vi "executePlayVSS.vi"(8 "error in (no error)":errorcluster, 11 "Game in":refnum<class "Game.lvclass">) -> (0 "error out":errorcluster, 3 "Game out":refnum<class "Game.lvclass">)   [LabVIEW 2023, in "Game.lvclass"]
uses:
  Game.lvclass
  Utilities_class/Utilities.lvclass
  Game.lvclass/Game.ctl
  Team_class/Team.lvclass/Team.ctl
  Playbook_class/Playbook.lvclass/Playbook.ctl
  HaltPlay_class/HaltPlay.lvclass/HaltPlay.ctl
  TimeoutPlay_class/TimeoutPlay.lvclass/TimeoutPlay.ctl
  PrepareFreeBallPlayVSS_class/PrepareFreeBallPlayVSS.lvclass
  PrepareGoalKickEnemyPlayVSS_class/PrepareGoalKickEnemyPlayVSS.lvclass
  PrepareGoalKickAllyPlayVSS_class/PrepareGoalKickAllyPlayVSS.lvclass
  PrepareKickoffEnemyPlay_class/PrepareKickoffEnemyPlay.lvclass
  PrepareKickoffAllyPlayVSS_class/PrepareKickoffAllyPlayVSS.lvclass
  PreparePenaltyEnemyPlayVSS_class/PreparePenaltyEnemyPlayVSS.lvclass
  PreparePenaltyAllyPlayVSS_class/PreparePenaltyAllyPlayVSS.lvclass
  Playbook_class/Read offensive_plays.vi
  HaltPlay_class/Read Roles.vi
  TimeoutPlay_class/Read Roles.vi
  Read KeeperTeam.vi
  Team_class/Read RobotRef.vi
  Team_class/Write RobotRef.vi
  Team_class/Write OffensivePlay Finished.vi
  Write KeeperTeam.vi
  Ally_class/Ally.lvclass
  C:/Users/roboi/Downloads/VSS_AI-Larc2023 - Copia (2)/Team_class/Team.lvclass
  Playbook_class/Playbook.lvclass
  Robot_class/Robot.lvclass
  Play_class/Play.lvclass
  TestPlay_class/TestPlay.lvclass
  EnemyPossessionAtEnemyFieldPlay_class/EnemyPossessionAtEnemyFieldPlay.lvclass
  EnemyPossessionAtOurFieldPlay_class/EnemyPossessionAtOurFieldPlay.lvclass
  NormalGamePlay_class/NormalGamePlay.lvclass
  IndirectEnemyPlay_class/IndirectEnemyPlay.lvclass
  PrepareKickoffAllyPlay_class/PrepareKickoffAllyPlay.lvclass
  KickPenaltyAllyPlay_class/KickPenaltyAllyPlay.lvclass
  PreparePenaltyAllyPlay_class/PreparePenaltyAllyPlay.lvclass
  DirectEnemyPlay_class/DirectEnemyPlay.lvclass
  PreparePenaltyEnemyPlay_class/PreparePenaltyEnemyPlay.lvclass
  BallOutOfFieldPlay_class/BallOutOfFieldPlay.lvclass
  StopOffensivePlay_class/StopOffensivePlay.lvclass
  PassPlay_class/PassPlay.lvclass
  DirectKickPlay_class/DirectKickPlay.lvclass
  HaltPlay_class/HaltPlay.lvclass
  PreparePassPlay_class/PreparePassPlay.lvclass
  PassToStriker_class/PassToStriker.lvclass
  PassTo2ndStriker_class/PassTo2ndStriker.lvclass
  SimplePass_class/SimplePass.lvclass
  PrepareRollToPassPlay_class/PrepareRollToPassPlay.lvclass
  PrepareDoublePassPlay_class/PrepareDoublePassPlay.lvclass
  TableWith2ndStrikerPlay_class/TableWith2ndStrikerPlay.lvclass
  TableWithStrikerPlay_class/TableWithStrikerPlay.lvclass
  HaltRole_class/HaltRole.lvclass
  DeadBallPlayVSS_class/DeadBallPlayVSS.lvclass
  NormalGamePlayVSS_class/NormalGamePlayVSS.lvclass
  BallChallengePlayVSS_class/BallChallengePlayVSS.lvclass
  PenaltyEnemyPlayVSS_class/PenaltyEnemyPlayVSS.lvclass
  TimeoutPlay_class/TimeoutPlay.lvclass
  KickPenaltyAllyPlayVSS_class/KickPenaltyAllyPlayVSS.lvclass
  PrepareKickoffEnemyPlayVSS_class/PrepareKickoffEnemyPlayVSS.lvclass
  FreeBallPlayVSS_class/FreeBallPlayVSS.lvclass
  GoalKickAllyPlayVSS_class/GoalKickAllyPlayVSS.lvclass
  GoalKickEnemyPlayVSS_class/GoalKickEnemyPlayVSS.lvclass
  KickoffAllyPlayVSS_class/KickoffAllyPlayVSS.lvclass
  KickoffEnemyPlayVSS_class/KickoffEnemyPlayVSS.lvclass
  StopPlayVSS_class/StopPlayVSS.lvclass
  AttackerAimGoalRoleVSS_class/AttackerAimGoalRoleVSS.lvclass
  BallChallengerAttackerRoleVSS_class/BallChallengerAttackerRoleVSS.lvclass
  KeeperRoleVSS_class/KeeperRoleVSS.lvclass
  NormalAttackerRoleVSS_class/NormalAttackerRoleVSS.lvclass
  DefenderAreaRoleVSS_class/DefenderAreaRoleVSS.lvclass
  GoAndKickRoleVSS_class/GoAndKickRoleVSS.lvclass
  GoalKickKeeperRoleVSS_class/GoalKickKeeperRoleVSS.lvclass
  TimeoutRole_class/TimeoutRole.lvclass
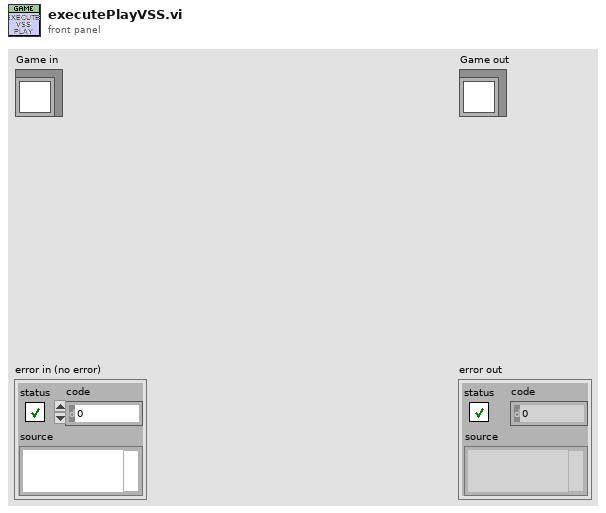
[diagram p1: front panel]
types:
  T1 = cluster{"id":i32, "x":dbl, "y":dbl, "orientation":dbl}[]
  T2 = enum16{"FreeBall", "PrepareFreeBall", "GoalKickEnemy", "GoalKickAlly", "KickoffAlly", "KickoffEnemy", "PrepareGoalKickEnemy", "PrepareGoalKickAlly", "Stop", "PrepareKickoffEnemy", "PrepareKickoffAlly", "PreparePenaltyEnemy", "Timeout", "DeadBall", "NormalGame", "KickPenaltyAlly", "PenaltyEnemy", "BallChallenge", "PreparePenaltyAlly", "Halt"}
  T3 = typedef "offensive_plays.ctl" = cluster{"Play":refnum<class "Play.lvclass">, "TestPlay":refnum<class "TestPlay.lvclass">, "EnemyPossessionAtEnemyFieldPlay":refnum<class "EnemyPossessionAtEnemyFieldPlay.lvclass">, "EnemyPossessionAtOurFieldPlay":refnum<class "EnemyPossessionAtOurFieldPlay.lvclass">, "NormalGamePlay":refnum<class "NormalGamePlay.lvclass">, "IndirectEnemyPlay":refnum<class "IndirectEnemyPlay.lvclass">, "PrepareKickoffAllyPlay":refnum<class "PrepareKickoffAllyPlay.lvclass">, "PrepareKickoffEnemyPlay":refnum<class "PrepareKickoffEnemyPlay.lvclass">, "KickPenaltyAllyPlay":refnum<class "KickPenaltyAllyPlay.lvclass">, "PreparePenaltyAllyPlay":refnum<class "PreparePenaltyAllyPlay.lvclass">, "DirectEnemyPlay":refnum<class "DirectEnemyPlay.lvclass">, "PreparePenaltyEnemyPlay":refnum<class "PreparePenaltyEnemyPlay.lvclass">, "BallOutOfFieldPlay":refnum<class "BallOutOfFieldPlay.lvclass">, "StopOffensivePlay":refnum<class "StopOffensivePlay.lvclass">, "PassPlay":refnum<class "PassPlay.lvclass">, "DirectKickPlay":refnum<class "DirectKickPlay.lvclass">, "HaltPlay":refnum<class "HaltPlay.lvclass">, "PreparePassPlay":refnum<class "PreparePassPlay.lvclass">, "PassToStrikerPlay":refnum<class "PassToStriker.lvclass">, "PassTo2ndStrikerPlay":refnum<class "PassTo2ndStriker.lvclass">, "SimplePassPlay":refnum<class "SimplePass.lvclass">, "PrepareRollToPassPlay":refnum<class "PrepareRollToPassPlay.lvclass">, "PrepareDoublePassPlay":refnum<class "PrepareDoublePassPlay.lvclass">, "TableWith2ndStrikerPlay":refnum<class "TableWith2ndStrikerPlay.lvclass">, "TableWithStrikerPlay":refnum<class "TableWithStrikerPlay.lvclass">}
  T4 = cluster{"HaltRole 1":refnum<class "HaltRole.lvclass">, "HaltRole 2":refnum<class "HaltRole.lvclass">, "HaltRole 3":refnum<class "HaltRole.lvclass">, "HaltRole 4":refnum<class "HaltRole.lvclass">, "HaltRole 5":refnum<class "HaltRole.lvclass">, "HaltRole 6":refnum<class "HaltRole.lvclass">}
  T5 = cluster{"PreparePenaltyAllyPlayVSS":refnum<class "PreparePenaltyAllyPlayVSS.lvclass">, "HaltPlay":refnum<class "HaltPlay.lvclass">, "DeadBallPlayVSS":refnum<class "DeadBallPlayVSS.lvclass">, "NormalGamePlayVSS":refnum<class "NormalGamePlayVSS.lvclass">, "BallChallengePlayVSS":refnum<class "BallChallengePlayVSS.lvclass">, "PenaltyEnemyPlayVSS":refnum<class "PenaltyEnemyPlayVSS.lvclass">, "TimeoutPlay":refnum<class "TimeoutPlay.lvclass">, "KickPenaltyAllyPlayVSS":refnum<class "KickPenaltyAllyPlayVSS.lvclass">, "PreparePenaltyEnemyPlayVSS":refnum<class "PreparePenaltyEnemyPlayVSS.lvclass">, "PrepareKickoffAllyPlayVSS":refnum<class "PrepareKickoffAllyPlayVSS.lvclass">, "PrepareKickoffEnemyPlayVSS":refnum<class "PrepareKickoffEnemyPlayVSS.lvclass">, "PrepareGoalKickAllyPlayVSS":refnum<class "PrepareGoalKickAllyPlayVSS.lvclass">, "PrepareGoalKickEnemyPlayVSS":refnum<class "PrepareGoalKickEnemyPlayVSS.lvclass">, "PrepareFreeBallPlayVSS":refnum<class "PrepareFreeBallPlayVSS.lvclass">, "FreeBallPlayVSS":refnum<class "FreeBallPlayVSS.lvclass">, "GoalKickAllyPlayVSS":refnum<class "GoalKickAllyPlayVSS.lvclass">, "GoalKickEnemyPlayVSS":refnum<class "GoalKickEnemyPlayVSS.lvclass">, "KickoffAllyPlayVSS":refnum<class "KickoffAllyPlayVSS.lvclass">, "KickoffEnemyPlayVSS":refnum<class "KickoffEnemyPlayVSS.lvclass">, "StopPlayVSS":refnum<class "StopPlayVSS.lvclass">}
  T6 = cluster{"HaltRole 1":refnum<class "HaltRole.lvclass">, "HaltRole 2":refnum<class "HaltRole.lvclass">, "AttackerAimGoalRoleVSS":refnum<class "AttackerAimGoalRoleVSS.lvclass">}
  T7 = cluster{"HaltRole 1":refnum<class "HaltRole.lvclass">, "HaltRole 2":refnum<class "HaltRole.lvclass">, "BallChallengerAttackerRoleVSS":refnum<class "BallChallengerAttackerRoleVSS.lvclass">}
  T8 = cluster{"KeeperRoleVSS":refnum<class "KeeperRoleVSS.lvclass">, "HaltRole A":refnum<class "HaltRole.lvclass">, "HaltRole D":refnum<class "HaltRole.lvclass">}
  T9 = cluster{"NormalAttackerRoleVSS":refnum<class "NormalAttackerRoleVSS.lvclass">, "HaltRole K":refnum<class "HaltRole.lvclass">, "HaltRole D":refnum<class "HaltRole.lvclass">}
  T10 = cluster{"NormalAttackerRoleVSS":refnum<class "NormalAttackerRoleVSS.lvclass">, "KeeperRoleVSS":refnum<class "KeeperRoleVSS.lvclass">, "DefenderAreaRoleVSS":refnum<class "DefenderAreaRoleVSS.lvclass">}
  T11 = cluster{"HaltRole K":refnum<class "HaltRole.lvclass">, "HaltRole D":refnum<class "HaltRole.lvclass">, "HaltRole A":refnum<class "HaltRole.lvclass">}
  T12 = cluster{"KeeperRoleVSS":refnum<class "KeeperRoleVSS.lvclass">, "HaltRole":refnum<class "HaltRole.lvclass">, "GoAndKickRoleVSS":refnum<class "GoAndKickRoleVSS.lvclass">}
  T13 = cluster{"HaltRole A":refnum<class "HaltRole.lvclass">, "HaltRole D":refnum<class "HaltRole.lvclass">, "GoalKickKeeperRoleVSS":refnum<class "GoalKickKeeperRoleVSS.lvclass">}
  T14 = cluster{"KeeperRoleVSS":refnum<class "KeeperRoleVSS.lvclass">, "DefenderAreaRoleVSS":refnum<class "DefenderAreaRoleVSS.lvclass">, "HaltRole":refnum<class "HaltRole.lvclass">}
  T15 = cluster{"TimeoutRole 1":refnum<class "TimeoutRole.lvclass">, "TimeoutRole 2":refnum<class "TimeoutRole.lvclass">, "TimeoutRole 3":refnum<class "TimeoutRole.lvclass">, "TimeoutRole 4":refnum<class "TimeoutRole.lvclass">, "TimeoutRole 5":refnum<class "TimeoutRole.lvclass">, "TimeoutRole 6":refnum<class "TimeoutRole.lvclass">}
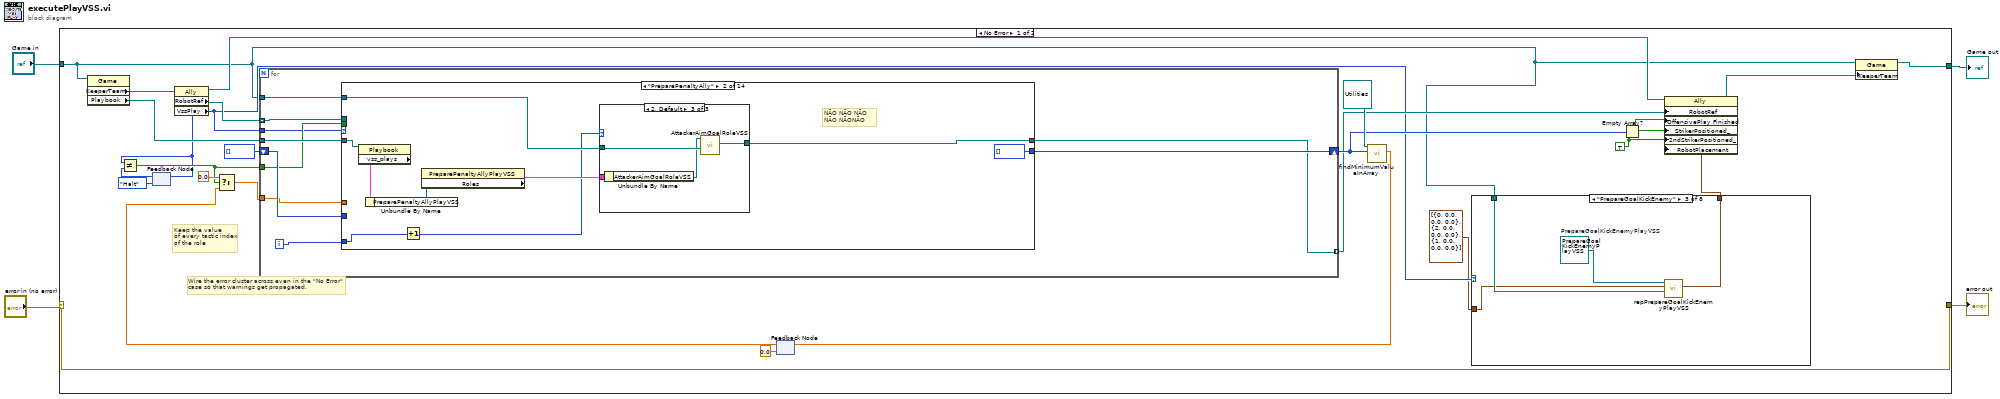
[diagram p0: block diagram]
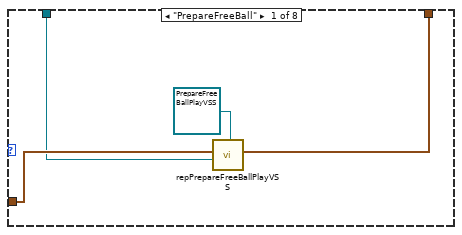
[diagram p2: hidden frame]
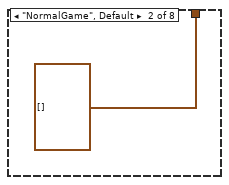
[diagram p3: hidden frame]
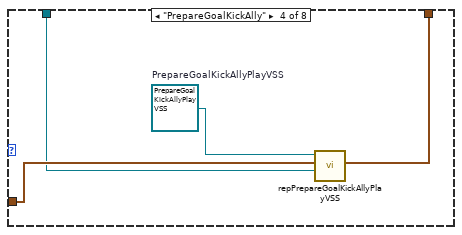
[diagram p4: hidden frame]
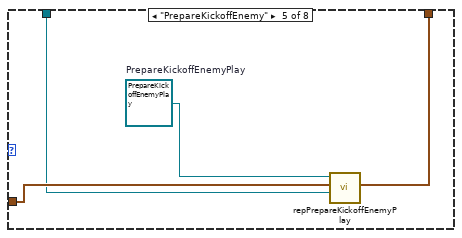
[diagram p5: hidden frame]
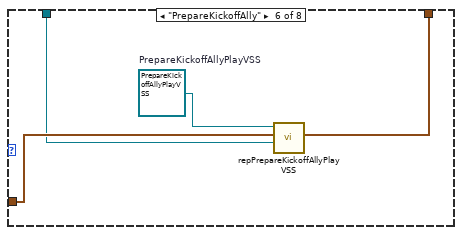
[diagram p6: hidden frame]
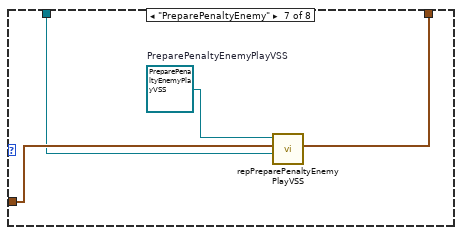
[diagram p7: hidden frame]
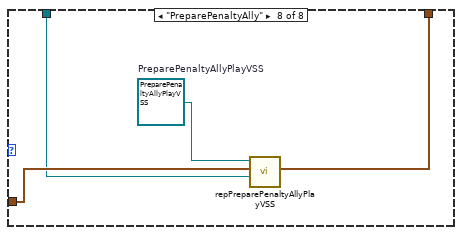
[diagram p8: hidden frame]
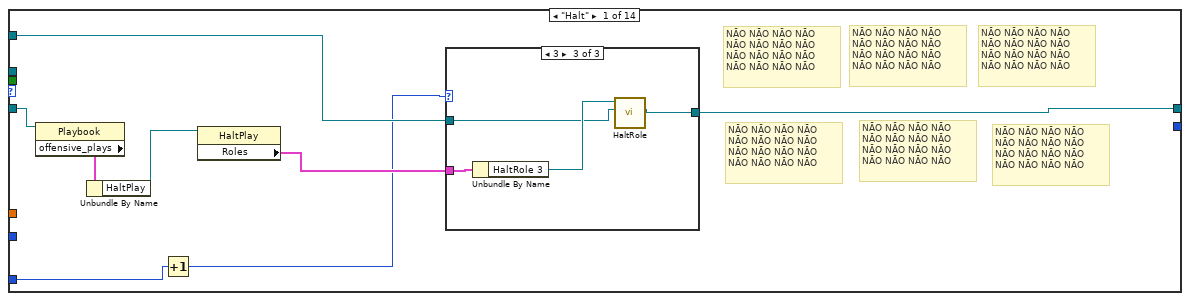
[diagram p9: hidden frame]
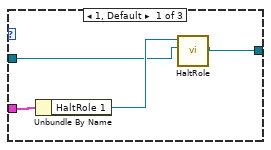
[diagram p10: hidden frame]
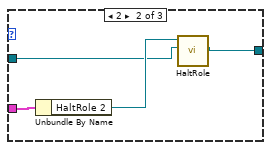
[diagram p11: hidden frame]
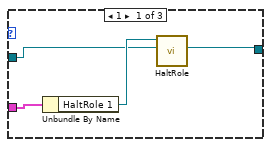
[diagram p12: hidden frame]
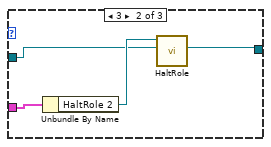
[diagram p13: hidden frame]
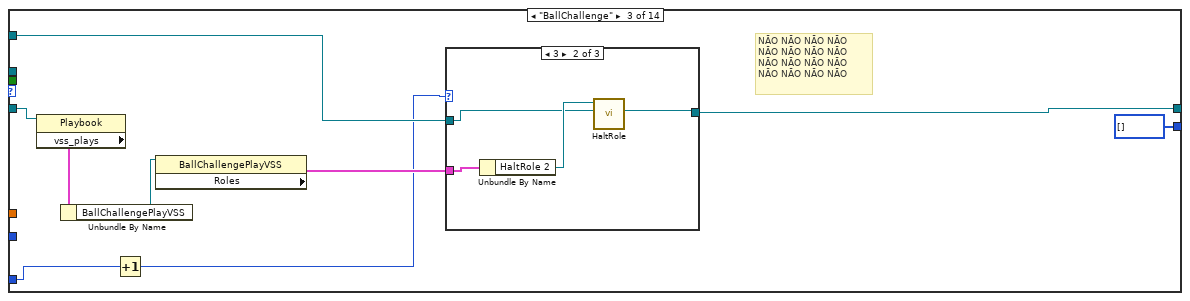
[diagram p14: hidden frame]
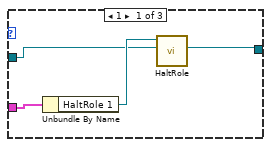
[diagram p15: hidden frame]
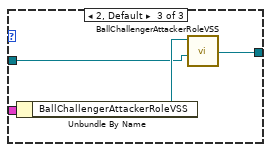
[diagram p16: hidden frame]
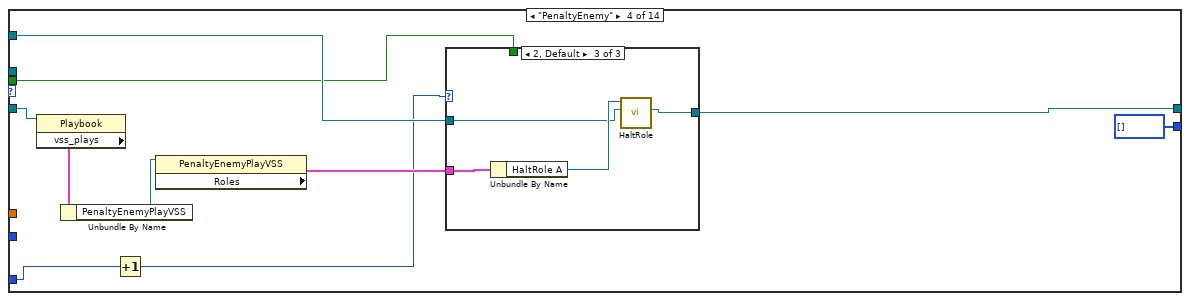
[diagram p17: hidden frame]
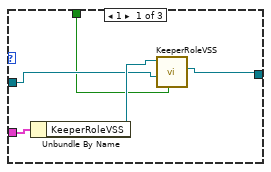
[diagram p18: hidden frame]
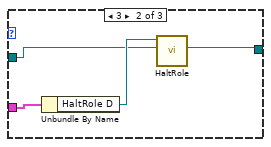
[diagram p19: hidden frame]
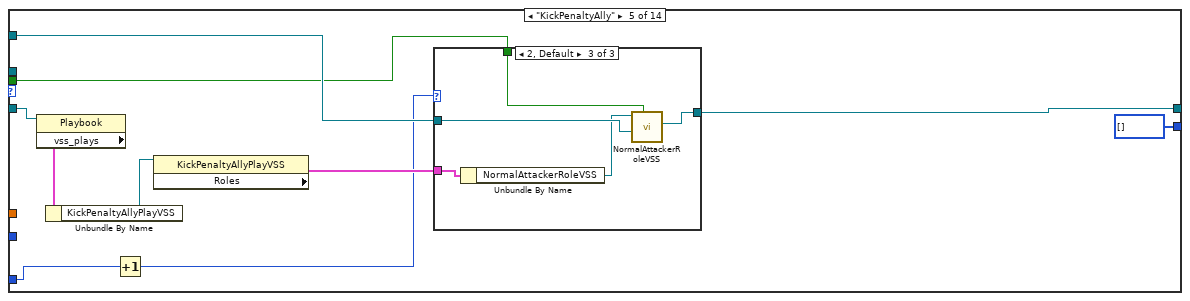
[diagram p20: hidden frame]
diagram:
  n1 = case shown="No Error" "error in (no error)" {
    selector: "error in (no error)" -> [w29 w389]
    tunnel: [w29 w389] -> w3
    tunnel: [w7 w388] -> w4
    tunnel: "Game in" -> [w8 w388]
    frame No Error {
      w14 = TRUE
      # "Keep the value\nof every tactic index\nof the role"
      # "Wire the error cluster across even in the \"No Error\"\ncase so that warnings get propagated."
      n2 = property class="Game"(reference=w8) -> ("KeeperTeam"=w28:refnum<class "Ally.lvclass">, "Playbook"=w26:refnum<class "Playbook.lvclass">)  [unwired: 1 in, 2 out]
      n3 = feedback #1(T2."Halt" ("VssPlay")) -> (w21:T2)
      n4 = property class="Ally"(reference=w28) -> (reference out=w12:refnum<class "Ally.lvclass">, "RobotRef"=w27:refnum<class "Robot.lvclass">[], "VssPlay"=w9:T2)  [unwired: 1 in, 1 out]
      n5 = Not Equal?(x=w9, y=w21) -> (x != y?=w18:bool)
      n6 = feedback-in #1(w9) -> ()
      n7 = feedback #2(0.0 ("minimum")) -> (w20:dbl)
      n8 = Select(t=0.0, s=w18, f=w20) -> (s? t:f=w13:dbl)
      n9 = for {
        tunnel: w27 -> [w63] mode=indexing
        tunnel: w26 -> [w68]
        tunnel: w8 -> [w67]
        shift-right: [w66] -> w16
        shift-left: i32[] [] -> [w65]
        tunnel: w18 -> [w64]
        tunnel: w13 -> [w62]
        tunnel: [w60] -> w11 mode=indexing
        tunnel: w9 -> [w59]
        i -> [w61]
        n10 = case shown="\"PreparePenaltyAlly\"" w59 {
          tunnel: w68 -> [w76 w97 w118 w140 w163 w186 w211 w233 w257 w280 w303 w328 w350 w372]
          tunnel: w67 -> [w72 w93 w114 w136 w159 w182 w207 w229 w253 w276 w299 w324 w346 w368]
          tunnel: [w71 w92 w113 w135 w158 w181 w206 w228 w252 w275 w298 w323 w345 w367] -> w60
          tunnel: w62 -> [_ _ _ _ _ _ _ _ _ _ _ _ _ _]
          tunnel: [_ i32[] [] i32[] [] i32[] [] i32[] [] i32[] [] i32[] [] i32[] [] i32[] [] i32[] [] i32[] [] i32[] [] i32[] [] i32[] []] -> w66
          tunnel: w65 -> [_ _ _ _ _ _ _ _ _ _ _ _ _ _]
          tunnel: w64 -> [_ _ _ w131 w154 w177 w202 w224 w248 w271 w294 w319 _ _]
          tunnel: w63 -> [_ _ _ _ _ _ _ _ _ _ _ _ _ w363]
          tunnel: w61 -> [w70 w90 w111 w133 w156 w179 w204 w226 w250 w273 w296 w321 w343 w365]
          frame "Halt" {
            # "NÃO NÃO NÃO NÃO\nNÃO NÃO NÃO NÃO\nNÃO NÃO NÃO NÃO\nNÃO NÃO NÃO NÃO"
            # "NÃO NÃO NÃO NÃO\nNÃO NÃO NÃO NÃO\nNÃO NÃO NÃO NÃO\nNÃO NÃO NÃO NÃO"
            # "NÃO NÃO NÃO NÃO\nNÃO NÃO NÃO NÃO\nNÃO NÃO NÃO NÃO\nNÃO NÃO NÃO NÃO"
            # "NÃO NÃO NÃO NÃO\nNÃO NÃO NÃO NÃO\nNÃO NÃO NÃO NÃO\nNÃO NÃO NÃO NÃO"
            # "NÃO NÃO NÃO NÃO\nNÃO NÃO NÃO NÃO\nNÃO NÃO NÃO NÃO\nNÃO NÃO NÃO NÃO"
            # "NÃO NÃO NÃO NÃO\nNÃO NÃO NÃO NÃO\nNÃO NÃO NÃO NÃO\nNÃO NÃO NÃO NÃO"
            n11 = property class="Playbook"(reference=w76) -> ("offensive_plays"=w75:T3)  [unwired: 1 in, 2 out]
            n12 = Unbundle By Name(w75) -> ("HaltPlay"=w74:refnum<class "HaltPlay.lvclass">)
            n13 = Increment(x=w70) -> (x+1=w69:i32)
            n14 = property class="HaltPlay"(reference=w74) -> ("Roles"=w73:T4)  [unwired: 1 in, 2 out]
            n15 = case shown="3" w69 {
              tunnel: w73 -> [w80 w84 w88]
              tunnel: w72 -> [w78 w82 w86]
              tunnel: [w77 w81 w85] -> w71
              frame 1, Default {
                n16 = Unbundle By Name(w80) -> ("HaltRole 1"=w79:refnum<class "HaltRole.lvclass">)
                n17 = call "HaltRole.vi"("Game in"=w78, "HaltRole in"=w79) -> ("Robot out"=w77:refnum<class "Robot.lvclass">)  [unwired: 6 in, 3 out]
              }
              frame 2 {
                n18 = Unbundle By Name(w84) -> ("HaltRole 2"=w83:refnum<class "HaltRole.lvclass">)
                n19 = call "HaltRole.vi"("Game in"=w82, "HaltRole in"=w83) -> ("Robot out"=w81:refnum<class "Robot.lvclass">)  [unwired: 6 in, 3 out]
              }
              frame 3 {
                n20 = Unbundle By Name(w88) -> ("HaltRole 3"=w87:refnum<class "HaltRole.lvclass">)
                n21 = call "HaltRole.vi"("Game in"=w86, "HaltRole in"=w87) -> ("Robot out"=w85:refnum<class "Robot.lvclass">)  [unwired: 6 in, 3 out]
              }
            }
          }
          frame "PreparePenaltyAlly" {
            # "NÃO NÃO NÃO \nNÃO NÃONÃO"
            n22 = property class="Playbook"(reference=w97) -> ("vss_plays"=w96:T5)  [unwired: 1 in, 2 out]
            n23 = Unbundle By Name(w96) -> ("PreparePenaltyAllyPlayVSS"=w95:refnum<class "PreparePenaltyAllyPlayVSS.lvclass">)
            n24 = Increment(x=w90) -> (x+1=w89:i32)
            n25 = property class="PreparePenaltyAllyPlayVSS"(reference=w95) -> ("Roles"=w94:T6)  [unwired: 1 in, 2 out]
            n26 = case shown="2, Default" w89 {
              tunnel: w94 -> [w101 w105 w109]
              tunnel: w93 -> [w99 w103 w107]
              tunnel: [w98 w102 w108] -> w92
              frame 1 {
                n27 = Unbundle By Name(w101) -> ("HaltRole 1"=w100:refnum<class "HaltRole.lvclass">)
                n28 = call "HaltRole.vi"("Game in"=w99, "HaltRole in"=w100) -> ("Robot out"=w98:refnum<class "Robot.lvclass">)  [unwired: 6 in, 3 out]
              }
              frame 3 {
                n29 = Unbundle By Name(w105) -> ("HaltRole 2"=w104:refnum<class "HaltRole.lvclass">)
                n30 = call "HaltRole.vi"("Game in"=w103, "HaltRole in"=w104) -> ("Robot out"=w102:refnum<class "Robot.lvclass">)  [unwired: 6 in, 3 out]
              }
              frame 2, Default {
                n31 = Unbundle By Name(w109) -> ("AttackerAimGoalRoleVSS"=w106:refnum<class "AttackerAimGoalRoleVSS.lvclass">)
                n32 = call "AttackerAimGoalRoleVSS.vi"("Game in"=w107, "AttackerAimGoalRoleVSS in"=w106) -> ("Robot out"=w108:refnum<class "Robot.lvclass">)  [unwired: 6 in, 3 out]
              }
            }
          }
          frame "BallChallenge" {
            # "NÃO NÃO NÃO NÃO\nNÃO NÃO NÃO NÃO\nNÃO NÃO NÃO NÃO\nNÃO NÃO NÃO NÃO"
            n33 = property class="Playbook"(reference=w118) -> ("vss_plays"=w117:T5)  [unwired: 1 in, 2 out]
            n34 = Unbundle By Name(w117) -> ("BallChallengePlayVSS"=w116:refnum<class "BallChallengePlayVSS.lvclass">)
            n35 = Increment(x=w111) -> (x+1=w110:i32)
            n36 = property class="BallChallengePlayVSS"(reference=w116) -> ("Roles"=w115:T7)  [unwired: 1 in, 2 out]
            n37 = case shown="3" w110 {
              tunnel: w115 -> [w122 w126 w130]
              tunnel: w114 -> [w120 w124 w127]
              tunnel: [w119 w123 w129] -> w113
              frame 1 {
                n38 = Unbundle By Name(w122) -> ("HaltRole 1"=w121:refnum<class "HaltRole.lvclass">)
                n39 = call "HaltRole.vi"("Game in"=w120, "HaltRole in"=w121) -> ("Robot out"=w119:refnum<class "Robot.lvclass">)  [unwired: 6 in, 3 out]
              }
              frame 3 {
                n40 = Unbundle By Name(w126) -> ("HaltRole 2"=w125:refnum<class "HaltRole.lvclass">)
                n41 = call "HaltRole.vi"("Game in"=w124, "HaltRole in"=w125) -> ("Robot out"=w123:refnum<class "Robot.lvclass">)  [unwired: 6 in, 3 out]
              }
              frame 2, Default {
                n42 = Unbundle By Name(w130) -> ("BallChallengerAttackerRoleVSS"=w128:refnum<class "BallChallengerAttackerRoleVSS.lvclass">)
                n43 = call "BallChallengerAttackerRoleVSS.vi"("Game in"=w127, "BallChallengerAttackerRoleVSS in"=w128) -> ("Robot out"=w129:refnum<class "Robot.lvclass">)  [unwired: 6 in, 3 out]
              }
            }
          }
          frame "PenaltyEnemy" {
            n44 = property class="Playbook"(reference=w140) -> ("vss_plays"=w139:T5)  [unwired: 1 in, 2 out]
            n45 = Unbundle By Name(w139) -> ("PenaltyEnemyPlayVSS"=w138:refnum<class "PenaltyEnemyPlayVSS.lvclass">)
            n46 = Increment(x=w133) -> (x+1=w132:i32)
            n47 = property class="PenaltyEnemyPlayVSS"(reference=w138) -> ("Roles"=w137:T8)  [unwired: 1 in, 2 out]
            n48 = case shown="2, Default" w132 {
              tunnel: w137 -> [w145 w149 w153]
              tunnel: w136 -> [w142 w147 w151]
              tunnel: [w144 w146 w150] -> w135
              tunnel: w131 -> [w141 _ _]
              frame 1 {
                n49 = Unbundle By Name(w145) -> ("KeeperRoleVSS"=w143:refnum<class "KeeperRoleVSS.lvclass">)
                n50 = call "KeeperRoleVSS.vi"("First call?"=w141, "Game in"=w142, "KeeperRoleVSS in"=w143) -> ("Robot out"=w144:refnum<class "Robot.lvclass">)  [unwired: 5 in, 3 out]
              }
              frame 3 {
                n51 = Unbundle By Name(w149) -> ("HaltRole D"=w148:refnum<class "HaltRole.lvclass">)
                n52 = call "HaltRole.vi"("Game in"=w147, "HaltRole in"=w148) -> ("Robot out"=w146:refnum<class "Robot.lvclass">)  [unwired: 6 in, 3 out]
              }
              frame 2, Default {
                n53 = Unbundle By Name(w153) -> ("HaltRole A"=w152:refnum<class "HaltRole.lvclass">)
                n54 = call "HaltRole.vi"("Game in"=w151, "HaltRole in"=w152) -> ("Robot out"=w150:refnum<class "Robot.lvclass">)  [unwired: 6 in, 3 out]
              }
            }
          }
          frame "KickPenaltyAlly" {
            n55 = property class="Playbook"(reference=w163) -> ("vss_plays"=w162:T5)  [unwired: 1 in, 2 out]
            n56 = Unbundle By Name(w162) -> ("KickPenaltyAllyPlayVSS"=w161:refnum<class "KickPenaltyAllyPlayVSS.lvclass">)
            n57 = Increment(x=w156) -> (x+1=w155:i32)
            n58 = property class="KickPenaltyAllyPlayVSS"(reference=w161) -> ("Roles"=w160:T9)  [unwired: 1 in, 2 out]
            n59 = case shown="2, Default" w155 {
              tunnel: w160 -> [w167 w171 w176]
              tunnel: w159 -> [w165 w169 w174]
              tunnel: [w164 w168 w172] -> w158
              tunnel: w154 -> [_ _ w175]
              frame 1 {
                n60 = Unbundle By Name(w167) -> ("HaltRole K"=w166:refnum<class "HaltRole.lvclass">)
                n61 = call "HaltRole.vi"("Game in"=w165, "HaltRole in"=w166) -> ("Robot out"=w164:refnum<class "Robot.lvclass">)  [unwired: 6 in, 3 out]
              }
              frame 3 {
                n62 = Unbundle By Name(w171) -> ("HaltRole D"=w170:refnum<class "HaltRole.lvclass">)
                n63 = call "HaltRole.vi"("Game in"=w169, "HaltRole in"=w170) -> ("Robot out"=w168:refnum<class "Robot.lvclass">)  [unwired: 6 in, 3 out]
              }
              frame 2, Default {
                n64 = Unbundle By Name(w176) -> ("NormalAttackerRoleVSS"=w173:refnum<class "NormalAttackerRoleVSS.lvclass">)
                n65 = call "NormalAttackerRoleVSS.vi"("First call?"=w175, "Game in"=w174, "NormalAttackerRoleVSS in"=w173) -> ("Robot out"=w172:refnum<class "Robot.lvclass">)  [unwired: 5 in, 3 out]
              }
            }
          }
          frame "NormalGame", Default {
            n66 = property class="Playbook"(reference=w186) -> ("vss_plays"=w185:T5)  [unwired: 1 in, 2 out]
            n67 = Unbundle By Name(w185) -> ("NormalGamePlayVSS"=w184:refnum<class "NormalGamePlayVSS.lvclass">)
            n68 = Increment(x=w179) -> (x+1=w178:i32)
            n69 = property class="NormalGamePlayVSS"(reference=w184) -> ("Roles"=w183:T10)  [unwired: 1 in, 2 out]
            n70 = case shown="2" w178 {
              tunnel: w183 -> [w191 w196 w201]
              tunnel: w182 -> [w189 w194 w199]
              tunnel: [w188 w193 w198] -> w181
              tunnel: w177 -> [w187 w192 w197]
              frame 1, Default {
                n71 = Unbundle By Name(w191) -> ("KeeperRoleVSS"=w190:refnum<class "KeeperRoleVSS.lvclass">)
                n72 = call "KeeperRoleVSS.vi"("First call?"=w187, "Game in"=w189, "KeeperRoleVSS in"=w190) -> ("Robot out"=w188:refnum<class "Robot.lvclass">)  [unwired: 5 in, 3 out]
              }
              frame 2 {
                n73 = Unbundle By Name(w196) -> ("NormalAttackerRoleVSS"=w195:refnum<class "NormalAttackerRoleVSS.lvclass">)
                n74 = call "NormalAttackerRoleVSS.vi"("First call?"=w192, "Game in"=w194, "NormalAttackerRoleVSS in"=w195) -> ("Robot out"=w193:refnum<class "Robot.lvclass">)  [unwired: 5 in, 3 out]
              }
              frame 3 {
                n75 = Unbundle By Name(w201) -> ("DefenderAreaRoleVSS"=w200:refnum<class "DefenderAreaRoleVSS.lvclass">)
                n76 = call "DefenderAreaRoleVSS.vi"("First call?"=w197, "Game in"=w199, "DefenderAreaRoleVSS in"=w200) -> ("Robot out"=w198:refnum<class "Robot.lvclass">)  [unwired: 5 in, 3 out]
              }
            }
          }
          frame "Stop" {
            n77 = property class="Playbook"(reference=w211) -> ("vss_plays"=w210:T5)  [unwired: 1 in, 2 out]
            n78 = Unbundle By Name(w210) -> ("StopPlayVSS"=w209:refnum<class "StopPlayVSS.lvclass">)
            n79 = Increment(x=w204) -> (x+1=w203:i32)
            n80 = property class="StopPlayVSS"(reference=w209) -> ("Roles"=w208:T11)  [unwired: 1 in, 2 out]
            n81 = case shown="2" w203 {
              tunnel: w208 -> [w215 w219 w223]
              tunnel: w207 -> [w214 w218 w222]
              tunnel: [w212 w216 w220] -> w206
              tunnel: w202 -> [_ _ _]
              frame 1, Default {
                n82 = Unbundle By Name(w215) -> ("HaltRole K"=w213:refnum<class "HaltRole.lvclass">)
                n83 = call "HaltRole.vi"("Game in"=w214, "HaltRole in"=w213) -> ("Robot out"=w212:refnum<class "Robot.lvclass">)  [unwired: 6 in, 3 out]
              }
              frame 3 {
                n84 = Unbundle By Name(w219) -> ("HaltRole D"=w217:refnum<class "HaltRole.lvclass">)
                n85 = call "HaltRole.vi"("Game in"=w218, "HaltRole in"=w217) -> ("Robot out"=w216:refnum<class "Robot.lvclass">)  [unwired: 6 in, 3 out]
              }
              frame 2 {
                n86 = Unbundle By Name(w223) -> ("HaltRole A"=w221:refnum<class "HaltRole.lvclass">)
                n87 = call "HaltRole.vi"("Game in"=w222, "HaltRole in"=w221) -> ("Robot out"=w220:refnum<class "Robot.lvclass">)  [unwired: 6 in, 3 out]
              }
            }
          }
          frame "KickoffAlly" {
            n88 = property class="Playbook"(reference=w233) -> ("vss_plays"=w232:T5)  [unwired: 1 in, 2 out]
            n89 = Unbundle By Name(w232) -> ("KickoffAllyPlayVSS"=w231:refnum<class "KickoffAllyPlayVSS.lvclass">)
            n90 = Increment(x=w226) -> (x+1=w225:i32)
            n91 = property class="KickoffAllyPlayVSS"(reference=w231) -> ("Roles"=w230:T12)  [unwired: 1 in, 2 out]
            n92 = case shown="2" w225 {
              tunnel: w230 -> [w238 w242 w247]
              tunnel: w229 -> [w236 w241 w245]
              tunnel: [w235 w239 w243] -> w228
              tunnel: w224 -> [w234 _ w246]
              frame 1, Default {
                n93 = Unbundle By Name(w238) -> ("KeeperRoleVSS"=w237:refnum<class "KeeperRoleVSS.lvclass">)
                n94 = call "KeeperRoleVSS.vi"("First call?"=w234, "Game in"=w236, "KeeperRoleVSS in"=w237) -> ("Robot out"=w235:refnum<class "Robot.lvclass">)  [unwired: 5 in, 3 out]
              }
              frame 3 {
                n95 = Unbundle By Name(w242) -> ("HaltRole"=w240:refnum<class "HaltRole.lvclass">)
                n96 = call "HaltRole.vi"("Game in"=w241, "HaltRole in"=w240) -> ("Robot out"=w239:refnum<class "Robot.lvclass">)  [unwired: 6 in, 3 out]
              }
              frame 2 {
                n97 = Unbundle By Name(w247) -> ("GoAndKickRoleVSS"=w244:refnum<class "GoAndKickRoleVSS.lvclass">)
                n98 = call "GoAndKickRoleVSS.vi"("First call?"=w246, "Game in"=w245, "GoAndKickRoleVSS in"=w244) -> ("Robot out"=w243:refnum<class "Robot.lvclass">)  [unwired: 5 in, 3 out]
              }
            }
          }
          frame "KickoffEnemy" {
            n99 = property class="Playbook"(reference=w257) -> ("vss_plays"=w256:T5)  [unwired: 1 in, 2 out]
            n100 = Unbundle By Name(w256) -> ("KickoffEnemyPlayVSS"=w255:refnum<class "KickoffEnemyPlayVSS.lvclass">)
            n101 = Increment(x=w250) -> (x+1=w249:i32)
            n102 = property class="KickoffEnemyPlayVSS"(reference=w255) -> ("Roles"=w254:T8)  [unwired: 1 in, 2 out]
            n103 = case shown="2" w249 {
              tunnel: w254 -> [w262 w266 w270]
              tunnel: w253 -> [w260 w265 w269]
              tunnel: [w259 w264 w267] -> w252
              tunnel: w248 -> [w258 _ _]
              frame 1, Default {
                n104 = Unbundle By Name(w262) -> ("KeeperRoleVSS"=w261:refnum<class "KeeperRoleVSS.lvclass">)
                n105 = call "KeeperRoleVSS.vi"("First call?"=w258, "Game in"=w260, "KeeperRoleVSS in"=w261) -> ("Robot out"=w259:refnum<class "Robot.lvclass">)  [unwired: 5 in, 3 out]
              }
              frame 3 {
                n106 = Unbundle By Name(w266) -> ("HaltRole D"=w263:refnum<class "HaltRole.lvclass">)
                n107 = call "HaltRole.vi"("Game in"=w265, "HaltRole in"=w263) -> ("Robot out"=w264:refnum<class "Robot.lvclass">)  [unwired: 6 in, 3 out]
              }
              frame 2 {
                n108 = Unbundle By Name(w270) -> ("HaltRole A"=w268:refnum<class "HaltRole.lvclass">)
                n109 = call "HaltRole.vi"("Game in"=w269, "HaltRole in"=w268) -> ("Robot out"=w267:refnum<class "Robot.lvclass">)  [unwired: 6 in, 3 out]
              }
            }
          }
          frame "GoalKickAlly" {
            n110 = property class="Playbook"(reference=w280) -> ("vss_plays"=w279:T5)  [unwired: 1 in, 2 out]
            n111 = Unbundle By Name(w279) -> ("GoalKickAllyPlayVSS"=w278:refnum<class "GoalKickAllyPlayVSS.lvclass">)
            n112 = Increment(x=w273) -> (x+1=w272:i32)
            n113 = property class="GoalKickAllyPlayVSS"(reference=w278) -> ("Roles"=w277:T13)  [unwired: 1 in, 2 out]
            n114 = case shown="2" w272 {
              tunnel: w277 -> [w285 w289 w293]
              tunnel: w276 -> [w282 w288 w292]
              tunnel: [w284 w287 w290] -> w275
              tunnel: w271 -> [w281 _ _]
              frame 1, Default {
                n115 = Unbundle By Name(w285) -> ("GoalKickKeeperRoleVSS"=w283:refnum<class "GoalKickKeeperRoleVSS.lvclass">)
                n116 = call "GoalKickKeeperRoleVSS.vi"("First call?"=w281, "Game in"=w282, "GoalKickKeeperRoleVSS in"=w283) -> ("Robot out"=w284:refnum<class "Robot.lvclass">)  [unwired: 5 in, 3 out]
              }
              frame 3 {
                n117 = Unbundle By Name(w289) -> ("HaltRole D"=w286:refnum<class "HaltRole.lvclass">)
                n118 = call "HaltRole.vi"("Game in"=w288, "HaltRole in"=w286) -> ("Robot out"=w287:refnum<class "Robot.lvclass">)  [unwired: 6 in, 3 out]
              }
              frame 2 {
                n119 = Unbundle By Name(w293) -> ("HaltRole A"=w291:refnum<class "HaltRole.lvclass">)
                n120 = call "HaltRole.vi"("Game in"=w292, "HaltRole in"=w291) -> ("Robot out"=w290:refnum<class "Robot.lvclass">)  [unwired: 6 in, 3 out]
              }
            }
          }
          frame "FreeBall" {
            n121 = property class="Playbook"(reference=w303) -> ("vss_plays"=w302:T5)  [unwired: 1 in, 2 out]
            n122 = Unbundle By Name(w302) -> ("FreeBallPlayVSS"=w301:refnum<class "FreeBallPlayVSS.lvclass">)
            n123 = Increment(x=w296) -> (x+1=w295:i32)
            n124 = property class="FreeBallPlayVSS"(reference=w301) -> ("Roles"=w300:T10)  [unwired: 1 in, 2 out]
            n125 = case shown="1, Default" w295 {
              tunnel: w300 -> [w308 w313 w318]
              tunnel: w299 -> [w306 w311 w316]
              tunnel: [w305 w310 w315] -> w298
              tunnel: w294 -> [w304 w309 w314]
              frame 1, Default {
                n126 = Unbundle By Name(w308) -> ("KeeperRoleVSS"=w307:refnum<class "KeeperRoleVSS.lvclass">)
                n127 = call "KeeperRoleVSS.vi"("First call?"=w304, "Game in"=w306, "KeeperRoleVSS in"=w307) -> ("Robot out"=w305:refnum<class "Robot.lvclass">)  [unwired: 5 in, 3 out]
              }
              frame 3 {
                n128 = Unbundle By Name(w313) -> ("DefenderAreaRoleVSS"=w312:refnum<class "DefenderAreaRoleVSS.lvclass">)
                n129 = call "DefenderAreaRoleVSS.vi"("First call?"=w309, "Game in"=w311, "DefenderAreaRoleVSS in"=w312) -> ("Robot out"=w310:refnum<class "Robot.lvclass">)  [unwired: 5 in, 3 out]
              }
              frame 2 {
                n130 = Unbundle By Name(w318) -> ("NormalAttackerRoleVSS"=w317:refnum<class "NormalAttackerRoleVSS.lvclass">)
                n131 = call "NormalAttackerRoleVSS.vi"("First call?"=w314, "Game in"=w316, "NormalAttackerRoleVSS in"=w317) -> ("Robot out"=w315:refnum<class "Robot.lvclass">)  [unwired: 5 in, 3 out]
              }
            }
          }
          frame "GoalKickEnemy" {
            n132 = property class="Playbook"(reference=w328) -> ("vss_plays"=w327:T5)  [unwired: 1 in, 2 out]
            n133 = Unbundle By Name(w327) -> ("GoalKickEnemyPlayVSS"=w326:refnum<class "GoalKickEnemyPlayVSS.lvclass">)
            n134 = Increment(x=w321) -> (x+1=w320:i32)
            n135 = property class="GoalKickEnemyPlayVSS"(reference=w326) -> ("Roles"=w325:T14)  [unwired: 1 in, 2 out]
            n136 = case shown="3" w320 {
              tunnel: w325 -> [w332 w337 w341]
              tunnel: w324 -> [w330 w335 w339]
              tunnel: [w329 w333 w338] -> w323
              tunnel: w319 -> [_ w336 _]
              frame 1, Default {
                n137 = Unbundle By Name(w332) -> ("KeeperRoleVSS"=w331:refnum<class "KeeperRoleVSS.lvclass">)
                n138 = call "KeeperRoleVSS.vi"("Game in"=w330, "KeeperRoleVSS in"=w331) -> ("Robot out"=w329:refnum<class "Robot.lvclass">)  [unwired: 6 in, 3 out]
              }
              frame 3 {
                n139 = Unbundle By Name(w337) -> ("DefenderAreaRoleVSS"=w334:refnum<class "DefenderAreaRoleVSS.lvclass">)
                n140 = call "DefenderAreaRoleVSS.vi"("First call?"=w336, "Game in"=w335, "DefenderAreaRoleVSS in"=w334) -> ("Robot out"=w333:refnum<class "Robot.lvclass">)  [unwired: 5 in, 3 out]
              }
              frame 2 {
                n141 = Unbundle By Name(w341) -> ("HaltRole"=w340:refnum<class "HaltRole.lvclass">)
                n142 = call "HaltRole.vi"("Game in"=w339, "HaltRole in"=w340) -> ("Robot out"=w338:refnum<class "Robot.lvclass">)  [unwired: 6 in, 3 out]
              }
            }
          }
          frame "DeadBall" {
            # "NÃO NÃO NÃO NÃO\nNÃO NÃO NÃO NÃO\nNÃO NÃO NÃO NÃO\nNÃO NÃO NÃO NÃO"
            n143 = property class="Playbook"(reference=w350) -> ("vss_plays"=w349:T5)  [unwired: 1 in, 2 out]
            n144 = Unbundle By Name(w349) -> ("DeadBallPlayVSS"=w348:refnum<class "DeadBallPlayVSS.lvclass">)
            n145 = Increment(x=w343) -> (x+1=w342:i32)
            n146 = property class="DeadBallPlayVSS"(reference=w348) -> ("Roles"=w347:T10)  [unwired: 1 in, 2 out]
            n147 = case shown="3" w342 {
              tunnel: w347 -> [w354 w358 w362]
              tunnel: w346 -> [w352 w356 w360]
              tunnel: [w351 w355 w359] -> w345
              frame 1 {
                n148 = Unbundle By Name(w354) -> ("KeeperRoleVSS"=w353:refnum<class "KeeperRoleVSS.lvclass">)
                n149 = call "KeeperRoleVSS.vi"("Game in"=w352, "KeeperRoleVSS in"=w353) -> ("Robot out"=w351:refnum<class "Robot.lvclass">)  [unwired: 6 in, 3 out]
              }
              frame 3 {
                n150 = Unbundle By Name(w358) -> ("DefenderAreaRoleVSS"=w357:refnum<class "DefenderAreaRoleVSS.lvclass">)
                n151 = call "DefenderAreaRoleVSS.vi"("Game in"=w356, "DefenderAreaRoleVSS in"=w357) -> ("Robot out"=w355:refnum<class "Robot.lvclass">)  [unwired: 6 in, 3 out]
              }
              frame 2, Default {
                n152 = Unbundle By Name(w362) -> ("NormalAttackerRoleVSS"=w361:refnum<class "NormalAttackerRoleVSS.lvclass">)
                n153 = call "NormalAttackerRoleVSS.vi"("Game in"=w360, "NormalAttackerRoleVSS in"=w361) -> ("Robot out"=w359:refnum<class "Robot.lvclass">)  [unwired: 6 in, 3 out]
              }
            }
          }
          frame "Timeout" {
            # "NÃO NÃO NÃO NÃO\nNÃO NÃO NÃO NÃO\nNÃO NÃO NÃO NÃO\nNÃO NÃO NÃO NÃO"
            n154 = property class="Playbook"(reference=w372) -> ("vss_plays"=w371:T5)  [unwired: 1 in, 2 out]
            n155 = Unbundle By Name(w371) -> ("TimeoutPlay"=w370:refnum<class "TimeoutPlay.lvclass">)
            n156 = Increment(x=w365) -> (x+1=w364:i32)
            n157 = property class="TimeoutPlay"(reference=w370) -> ("Roles"=w369:T15)  [unwired: 1 in, 2 out]
            n158 = case shown="2" w364 {
              tunnel: w369 -> [w377 w382 w387]
              tunnel: w368 -> [w375 w380 w385]
              tunnel: [w374 w379 w384] -> w367
              tunnel: w363 -> [w373 w378 w383]
              frame 1, Default {
                n159 = Unbundle By Name(w377) -> ("TimeoutRole 1"=w376:refnum<class "TimeoutRole.lvclass">)
                n160 = call-dynamic "TimeoutRole.vi"("Game in"=w375, "Robot in"=w373, "TimeoutRole in"=w376) -> ("Robot out"=w374:refnum<class "Robot.lvclass">)  [unwired: 5 in, 3 out]
              }
              frame 2 {
                n161 = Unbundle By Name(w382) -> ("TimeoutRole 2"=w381:refnum<class "TimeoutRole.lvclass">)
                n162 = call-dynamic "TimeoutRole.vi"("Game in"=w380, "Robot in"=w378, "TimeoutRole in"=w381) -> ("Robot out"=w379:refnum<class "Robot.lvclass">)  [unwired: 5 in, 3 out]
              }
              frame 3 {
                n163 = Unbundle By Name(w387) -> ("TimeoutRole 3"=w386:refnum<class "TimeoutRole.lvclass">)
                n164 = call-dynamic "TimeoutRole.vi"("Game in"=w385, "Robot in"=w383, "TimeoutRole in"=w386) -> ("Robot out"=w384:refnum<class "Robot.lvclass">)  [unwired: 5 in, 3 out]
              }
            }
          }
        }
      }
      n165 = call-dynamic "findMinimumValueInArray.vi"("array"=w16, "Utilities in"=refnum<class "Utilities.lvclass"> refnum) -> ("minimum"=w23:dbl)  [unwired: 7 in, 2 out]
      n166 = feedback-in #2(w23) -> ()
      n167 = case shown="\"PrepareGoalKickEnemy\"" w9 {
        tunnel: w8 -> [w30 _ w36 w41 w43 w48 w53 w56]
        tunnel: [w31 T1 [] ("RobotPlacement") w37 w39 w45 w47 w51 w55] -> w5
        tunnel: T1 [{"id"=0, "x"=0.0, "y"=0.0, "orientation"=0.0}, {"id"=2, "x"=0.0, "y"=0.0, "orientation"=0.0}, {"id"=1, "x"=0.0, "y"=0.0, "orientation"=0.0}] ("RobotPlacement") -> [w32 _ w35 w42 w44 w49 w54 w57]
        frame "PrepareFreeBall" {
          n168 = call "repPrepareFreeBallPlayVSS.vi"("Game in 2"=w30, "RobotPlacement"=w32, "PrepareFreeBallPlayVSS in"=refnum<class "PrepareFreeBallPlayVSS.lvclass"> refnum) -> ("RobotPlacement 2"=w31:T1)  [unwired: 6 in, 2 out]
        }
        frame "NormalGame", Default {
        }
        frame "PrepareGoalKickEnemy" {
          w38 = refnum<class "PrepareGoalKickEnemyPlayVSS.lvclass"> refnum  # PrepareGoalKickEnemyPlayVSS
          n169 = call "repPrepareGoalKickEnemyPlayVSS.vi"("PrepareGoalKickEnemyPlayVSS in"=w38, "RobotPlacement"=w35, "Game in 2"=w36) -> ("RobotPlacement 2"=w37:T1)  [unwired: 5 in, 2 out]
        }
        frame "PrepareGoalKickAlly" {
          w40 = refnum<class "PrepareGoalKickAllyPlayVSS.lvclass"> refnum  # PrepareGoalKickAllyPlayVSS
          n170 = call "repPrepareGoalKickAllyPlayVSS.vi"("Game in 2"=w41, "RobotPlacement"=w42, "PrepareGoalKickAllyPlayVSS in"=w40) -> ("RobotPlacement 2"=w39:T1)  [unwired: 6 in, 2 out]
        }
        frame "PrepareKickoffEnemy" {
          w46 = refnum<class "PrepareKickoffEnemyPlay.lvclass"> refnum  # PrepareKickoffEnemyPlay
          n171 = call "repPrepareKickoffEnemyPlay.vi"("Game in 2"=w43, "RobotPlacement"=w44, "PrepareKickoffEnemyPlay in"=w46) -> ("RobotPlacement 2"=w45:T1)  [unwired: 6 in, 2 out]
        }
        frame "PrepareKickoffAlly" {
          w50 = refnum<class "PrepareKickoffAllyPlayVSS.lvclass"> refnum  # PrepareKickoffAllyPlayVSS
          n172 = call "repPrepareKickoffAllyPlayVSS.vi"("Game in 2"=w48, "RobotPlacement"=w49, "PrepareKickoffAllyPlayVSS in"=w50) -> ("RobotPlacement 2"=w47:T1)  [unwired: 6 in, 2 out]
        }
        frame "PreparePenaltyEnemy" {
          w52 = refnum<class "PreparePenaltyEnemyPlayVSS.lvclass"> refnum  # PreparePenaltyEnemyPlayVSS
          n173 = call "repPreparePenaltyEnemyPlayVSS.vi"("Game in 2"=w53, "RobotPlacement"=w54, "PreparePenaltyEnemyPlayVSS in"=w52) -> ("RobotPlacement 2"=w51:T1)  [unwired: 6 in, 2 out]
        }
        frame "PreparePenaltyAlly" {
          w58 = refnum<class "PreparePenaltyAllyPlayVSS.lvclass"> refnum  # PreparePenaltyAllyPlayVSS
          n174 = call "repPreparePenaltyAllyPlayVSS.vi"("Game in 2"=w56, "RobotPlacement"=w57, "PreparePenaltyAllyPlayVSS in"=w58) -> ("RobotPlacement 2"=w55:T1)  [unwired: 6 in, 2 out]
        }
      }
      n175 = Empty Array?(array=w16) -> (empty?=w17:bool)
      n176 = property class="Ally"(reference=w12, "RobotRef"=w11, "OffensivePlay Finished"=w17, "StrikerPositioned_"=w14, "2ndStrikerPositioned_"=w14, "RobotPlacement"=w5) -> (reference out=w25:refnum<class "Ally.lvclass">)  [unwired: 1 in, 1 out]
      n177 = property class="Game"(reference=w8, "KeeperTeam"=w25) -> (reference out=w7:refnum<class "Game.lvclass">)  [unwired: 1 in, 1 out]
    }
    frame Error {
    }
  }
  "error out" <- w3
  "Game out" <- w4
